vi "run.vi"(8 "error in (no error)":errorcluster) -> (0 "error out":errorcluster)   [LabVIEW 2010, in "CPUmonitor.lvclass"]
uses:
  CPUmonitor.lvclass
  class_data.vi
panel:
  in  "slider":refnum<vi>
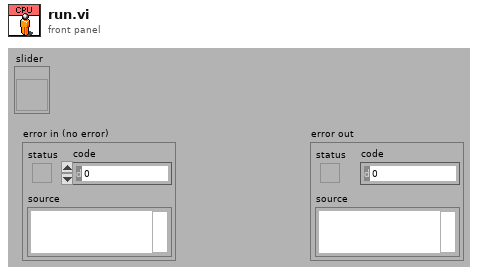
[diagram p1: front panel]
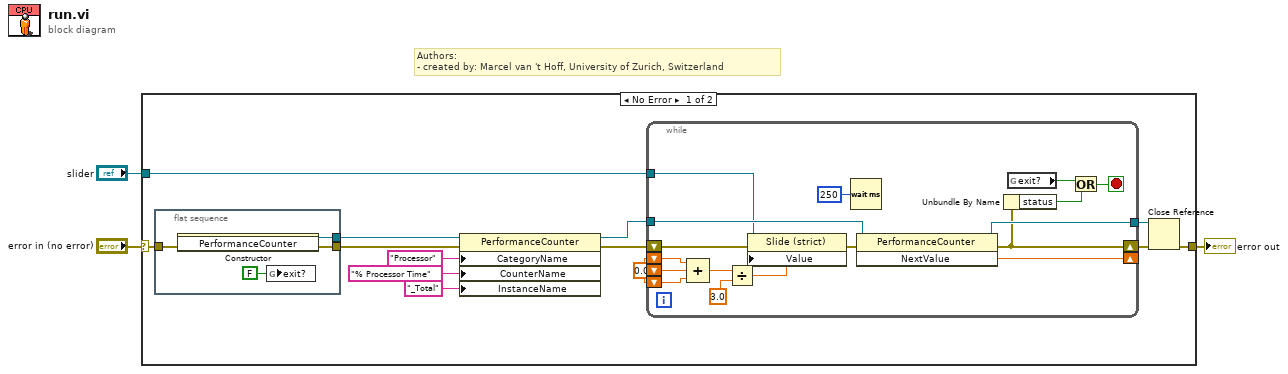
[diagram p0: block diagram]
diagram:
  # "Authors: \n- created by: Marcel van 't Hoff, University of Zurich, Switzerland"
  n1 = case shown="No Error" "error in (no error)" {
    selector: "error in (no error)" -> [w5 w38]
    tunnel: [w7 w38] -> w3
    tunnel: "slider" -> [w4 _]
    frame No Error {
      w6 = sgl 0.0 ("NextValue")
      n2 = flat-sequence {
        tunnel: [w20] -> w16
        tunnel: [w19] -> w12
        tunnel: w5 -> [w18]
        frame #0 {
          n3 = constructor class="PerformanceCounter"(error in=w18) -> (reference out=w20:refnum<k24>, error out=w19:errorcluster)  [unwired: 2 in, 1 out]
          n4 = global write "class_data.vi" "exit?"(FALSE ("exit?")) -> ()
        }
      }
      n5 = property class="PerformanceCounter"(reference=w16, error in=w12, "CategoryName"="Processor", "CounterName"="% Processor Time", "InstanceName"="_Total") -> (reference out=w11:refnum<k24>, error out=w10:errorcluster)
      n6 = while {
        tunnel: w11 -> [w37]
        tunnel: [w36] -> w9
        shift-right: [w23] -> w8
        shift-left: w10 -> [w25]
        shift-right: [w35] -> _
        shift-left: w6 -> [w33]
        shift-left: w6 -> [w32]
        shift-left: w6 -> [w29]
        tunnel: w4 -> [w21]
        stop <- w27 stop-if-true
        n7 = Compound Arithmetic op=ADD(w33, w32, w29) -> (w31:sgl)
        n8 = Divide(x=w31, y=sgl 3.0) -> (x/y=w26:sgl)
        n9 = property class="Slide (strict)"(reference=w21, error in=w25, "Value"=w26) -> (error out=w24:errorcluster)  [unwired: 1 out]
        n10 = Wait (ms)(milliseconds to wait=u32 250) -> ()  [unwired: 1 out]
        n11 = invoke class="PerformanceCounter" method="NextValue"(reference=w37, error in=w24) -> (reference out=w36:refnum<k24>, error out=w23:errorcluster, "NextValue"=w35:sgl)  [unwired: 1 in]
        n12 = Unbundle By Name(w23) -> ("status"=w28:bool)
        n13 = global read "class_data.vi" "exit?"() -> (w22:bool)
        n14 = Or(x=w22, y=w28) -> (x .or. y?=w27:bool)
      }
      n15 = Close Reference(reference=w9, error in (no error)=w8) -> (error out=w7:errorcluster)
    }
    frame Error {
    }
  }
  "error out" <- w3
